vi "Get Static.vi"(8 "error in (no error)":errorcluster, 11 "Splitter in":refnum<class "Splitter.lvclass">) -> (0 "error out":errorcluster, 2 "Static?":bool, 3 "Splitter out":refnum<class "Splitter.lvclass">)   [LabVIEW 2013, in "Splitter.lvclass"]
doc: "Copyright 2018, Wiebe Walstra, wiebe@carya.nl."
uses:
  Splitter.lvclass
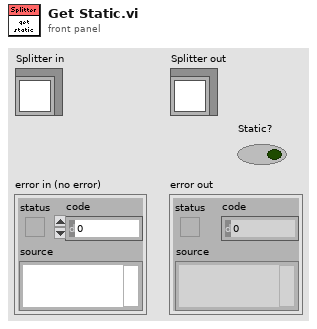
[diagram p1: front panel]
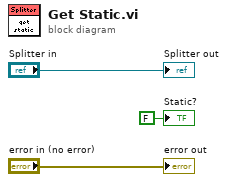
[diagram p0: block diagram]
diagram:
  "error out" <- "error in (no error)"
  "Splitter out" <- "Splitter in"
  "Static?" <- FALSE ("Static?")
